vi "Read CarWash Constants.vi"(8 "error in":errorcluster, 11 "CFG File Refnum in":T2) -> (0 "error out":errorcluster, 3 "CFG File Refnum out":T2)   [LabVIEW 2017]
uses:
  <vilib>/Utility/config.llb/Config Data RefNum.ctl
  Configuration Data.ctl
  <vilib>/Utility/config.llb/Read Key (U32).vi
  <vilib>/Utility/error.llb/Error Cluster From Error Code.vi
  <vilib>/ErrorRing/Error Ring.xnode
  <vilib>/Utility/config.llb/NI_LVConfig.lvlib
panel:
  out "Cluster":T1
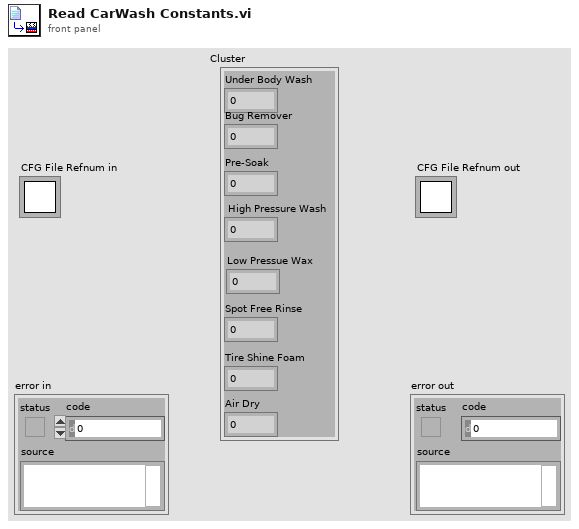
[diagram p1: front panel]
types:
  T1 = typedef "Configuration Data.ctl" = cluster{"Under Body Wash ":u32, "Bug Remover":u32, "Pre-Soak":u32, " High Pressure Wash":u32, "Low Pressue Wax ":u32, "Spot Free Rinse ":u32, "Tire Shine Foam":u32, "Air Dry ":u32}
  T2 = typedef "NI_LVConfig.lvlib/Config Data RefNum.ctl" = refnum<k1>
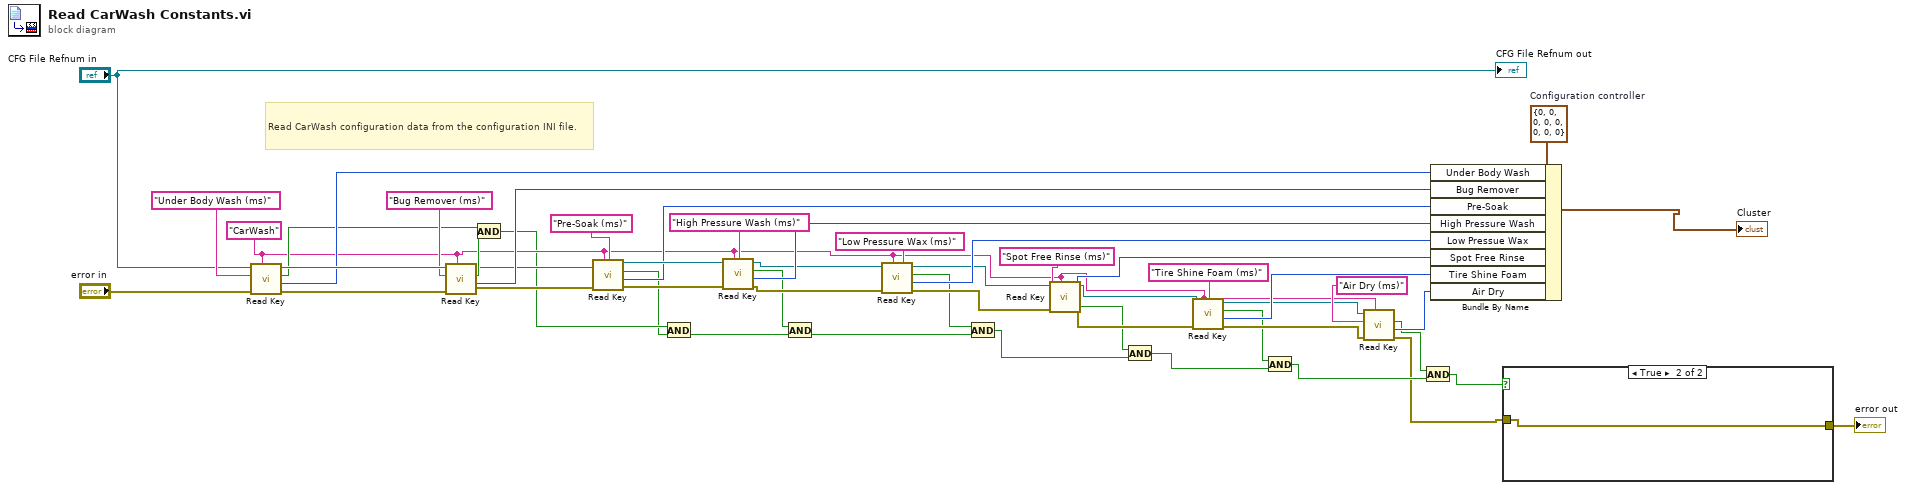
[diagram p0: block diagram]
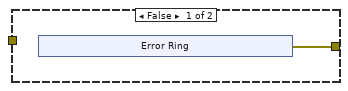
[diagram p2: hidden frame]
diagram:
  w42 = T1 {"Under Body Wash "=0, "Bug Remover"=0, "Pre-Soak"=0, " High Pressure Wash"=0, "Low Pressue Wax "=0, "Spot Free Rinse "=0, "Tire Shine Foam"=0, "Air Dry "=0}  # Configuration controller
  w20 = "CarWash" ("section")
  # "Read CarWash configuration data from the configuration INI file."
  n1 = call-poly <vilib>:"Read Key.vi"("section"=w20, "error in (no error)"="error in", "key"="Under Body Wash (ms)", "refnum"="CFG File Refnum in") -> ("error out"=w51:errorcluster, "value"=w47:u32, "found?"=w43:bool, "refnum out"=w50:T2)  [unwired: 4 in]
  n2 = call-poly <vilib>:"Read Key.vi"("section"=w20, "error in (no error)"=w51, "key"="Bug Remover (ms)", "refnum"=w50) -> ("error out"=w39:errorcluster, "value"=w46:u32, "found?"=w44:bool, "refnum out"=w40:T2)  [unwired: 4 in]
  n3 = And(x=w43, y=w44) -> (x .and. y?=w15:bool)
  n4 = call-poly <vilib>:"Read Key.vi"("section"=w20, "error in (no error)"=w39, "key"="Pre-Soak (ms)", "refnum"=w40) -> ("error out"=w37:errorcluster, "value"=w35:u32, "found?"=w14:bool, "refnum out"=w36:T2)  [unwired: 4 in]
  n5 = And(x=w15, y=w14) -> (x .and. y?=w12:bool)
  n6 = call-poly <vilib>:"Read Key.vi"("section"=w20, "error in (no error)"=w37, "key"="High Pressure Wash (ms)", "refnum"=w36) -> ("error out"=w32:errorcluster, "value"=w34:u32, "found?"=w13:bool, "refnum out"=w31:T2)  [unwired: 4 in]
  n7 = And(x=w13, y=w12) -> (x .and. y?=w10:bool)
  n8 = call-poly <vilib>:"Read Key.vi"("section"=w20, "error in (no error)"=w32, "key"="Low Pressure Wax (ms)", "refnum"=w31) -> ("error out"=w28:errorcluster, "value"=w30:u32, "found?"=w11:bool, "refnum out"=w27:T2)  [unwired: 4 in]
  n9 = And(x=w11, y=w10) -> (x .and. y?=w8:bool)
  n10 = call-poly <vilib>:"Read Key.vi"("section"=w20, "error in (no error)"=w28, "key"="Spot Free Rinse (ms)", "refnum"=w27) -> ("error out"=w23:errorcluster, "value"=w24:u32, "found?"=w9:bool, "refnum out"=w22:T2)  [unwired: 4 in]
  n11 = And(x=w9, y=w8) -> (x .and. y?=w6:bool)
  n12 = call-poly <vilib>:"Read Key.vi"("section"=w20, "error in (no error)"=w23, "key"="Tire Shine Foam (ms)", "refnum"=w22) -> ("error out"=w19:errorcluster, "value"=w21:u32, "found?"=w7:bool, "refnum out"=w18:T2)  [unwired: 4 in]
  n13 = And(x=w7, y=w6) -> (x .and. y?=w5:bool)
  n14 = call-poly <vilib>:"Read Key.vi"("section"=w20, "error in (no error)"=w19, "key"="Air Dry (ms)", "refnum"=w18) -> ("error out"=w2:errorcluster, "value"=w17:u32, "found?"=w4:bool)  [unwired: 4 in, 1 out]
  n15 = And(x=w4, y=w5) -> (x .and. y?=w3:bool)
  n16 = Bundle By Name(cluster=w42, "Under Body Wash"=w47, "Bug Remover"=w46, "Pre-Soak"=w35, "High Pressure Wash"=w34, "Low Pressue Wax"=w30, "Spot Free Rinse"=w24, "Tire Shine Foam"=w21, "Air Dry"=w17) -> (→"Cluster":T1)
  n17 = case shown="True" w3 {
    tunnel: [w53 w59] -> w45
    tunnel: w2 -> [_ w59]
    frame False {
      n18 = xnode "Error Ring"() -> ("error out"=w53:errorcluster)
    }
    frame True {
    }
  }
  "error out" <- w45
  "CFG File Refnum out" <- "CFG File Refnum in"
